vi "CaliperCheckResultDifference.vi"(10 "New Result":T1, 11 "Old Result":T1) -> (2 "ResultDiff?":bool)   [LabVIEW 2019]
uses:
  Controls/CaliperResult.ctl
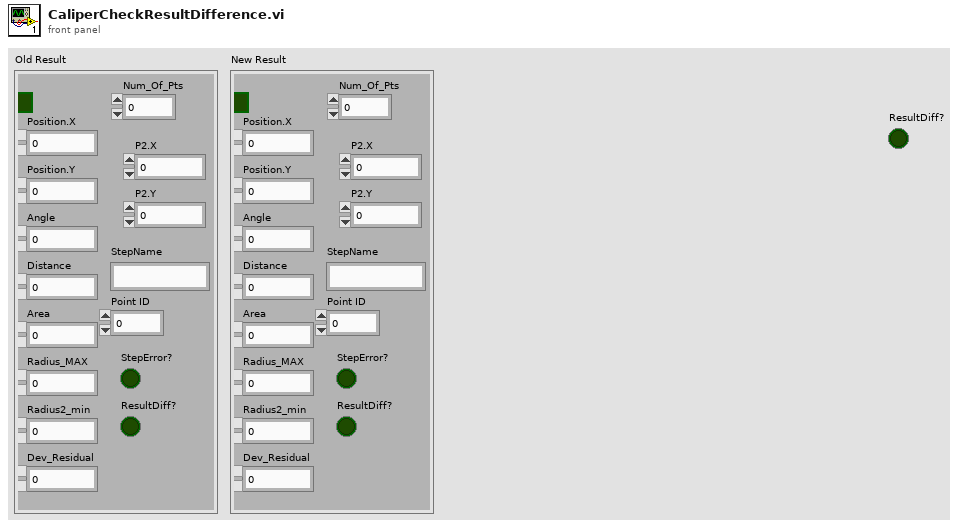
[diagram p1: front panel]
types:
  T1 = typedef "CaliperResult.ctl" = cluster{"PointInclude?":bool, "Num_Of_Pts":u8, "Position.X":dbl, "Position.Y":dbl, "Angle":dbl, "Distance":dbl, "Area":dbl, "Radius_MAX":dbl, "Radius2_min":dbl, "Dev_Residual":dbl, "P2.X":dbl, "P2.Y":dbl, "StepName":string, "Point ID":u8, "StepError?":bool, "ResultDiff?":bool}
  T2 = cluster{"Position.X":dbl, "Position.Y":dbl, "Angle":dbl, "Distance":dbl, "Area":dbl, "Radius_MAX":dbl, "Radius2_min":dbl, "Dev_Residual":dbl, "P2.X":dbl, "P2.Y":dbl}
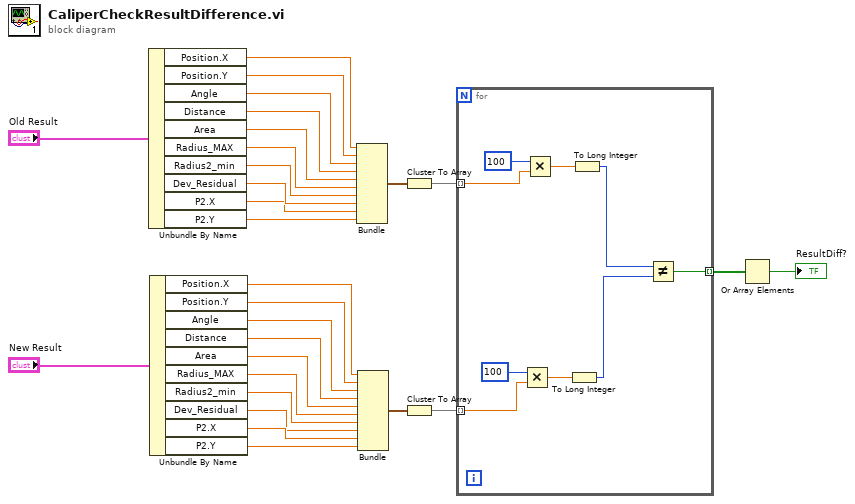
[diagram p0: block diagram]
diagram:
  n1 = Unbundle By Name("Old Result") -> ("Position.X"=w27:dbl, "Position.Y"=w26:dbl, "Angle"=w25:dbl, "Distance"=w24:dbl, "Area"=w23:dbl, "Radius_MAX"=w22:dbl, "Radius2_min"=w21:dbl, "Dev_Residual"=w20:dbl, "P2.X"=w19:dbl, "P2.Y"=w18:dbl)
  n2 = Unbundle By Name("New Result") -> ("Position.X"=w8:dbl, "Position.Y"=w9:dbl, "Angle"=w10:dbl, "Distance"=w11:dbl, "Area"=w12:dbl, "Radius_MAX"=w13:dbl, "Radius2_min"=w14:dbl, "Dev_Residual"=w15:dbl, "P2.X"=w16:dbl, "P2.Y"=w17:dbl)
  n3 = Bundle("Position.X"=w27, "Position.Y"=w26, "Angle"=w25, "Distance"=w24, "Area"=w23, "Radius_MAX"=w22, "Radius2_min"=w21, "Dev_Residual"=w20, "P2.X"=w19, "P2.Y"=w18) -> (w6:T2)  [unwired: 1 in]
  n4 = Bundle("Position.X"=w8, "Position.Y"=w9, "Angle"=w10, "Distance"=w11, "Area"=w12, "Radius_MAX"=w13, "Radius2_min"=w14, "Dev_Residual"=w15, "P2.X"=w16, "P2.Y"=w17) -> (w5:T2)  [unwired: 1 in]
  n5 = Cluster To Array(cluster=w6) -> (array=w4:dbl[])
  n6 = Cluster To Array(cluster=w5) -> (array=w3:dbl[])
  n7 = for {
    tunnel: w4 -> [w32] mode=indexing
    tunnel: w3 -> [w33] mode=indexing
    tunnel: [w29] -> w2 mode=indexing
    n8 = Multiply(x=100, y=w33) -> (x*y=w35:dbl)
    n9 = Multiply(x=100, y=w32) -> (x*y=w37:dbl)
    n10 = To Long Integer(number=w35) -> (32bit integer=w30:i32)
    n11 = To Long Integer(number=w37) -> (32bit integer=w31:i32)
    n12 = Not Equal?(x=w31, y=w30) -> (x != y?=w29:bool)
  }
  n13 = Or Array Elements(Boolean array=w2) -> (logical OR=→"ResultDiff?":bool)
